vi "Get Test Limits File Path.vi"(6 "Lookup Table File Name":string="TestLimitsLookup.csv", 8 "error in (no error)":errorcluster, 9 "Filename Search Parameters":string, 10 "HW Version":dbl, 11 "Test Limits Directory":path) -> (0 "error out":errorcluster, 3 "Test Limits File Path":path)   [LabVIEW 2025, in "Test Limits.lvlib"]
uses:
  Test Limits.lvlib
  <vilib>/Utility/error.llb/Error Cluster From Error Code.vi
  <vilib>/ErrorRing/Error Ring.xnode
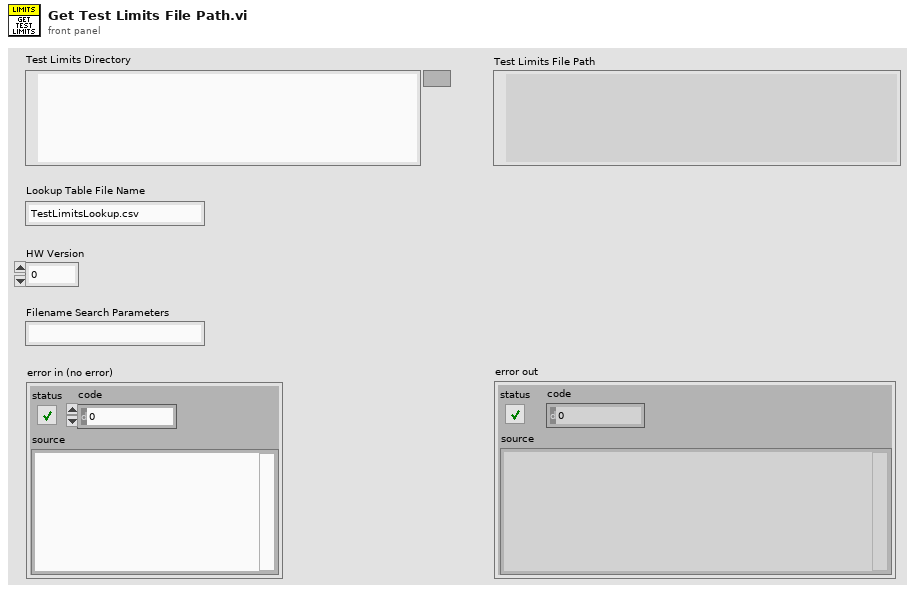
[diagram p1: front panel]
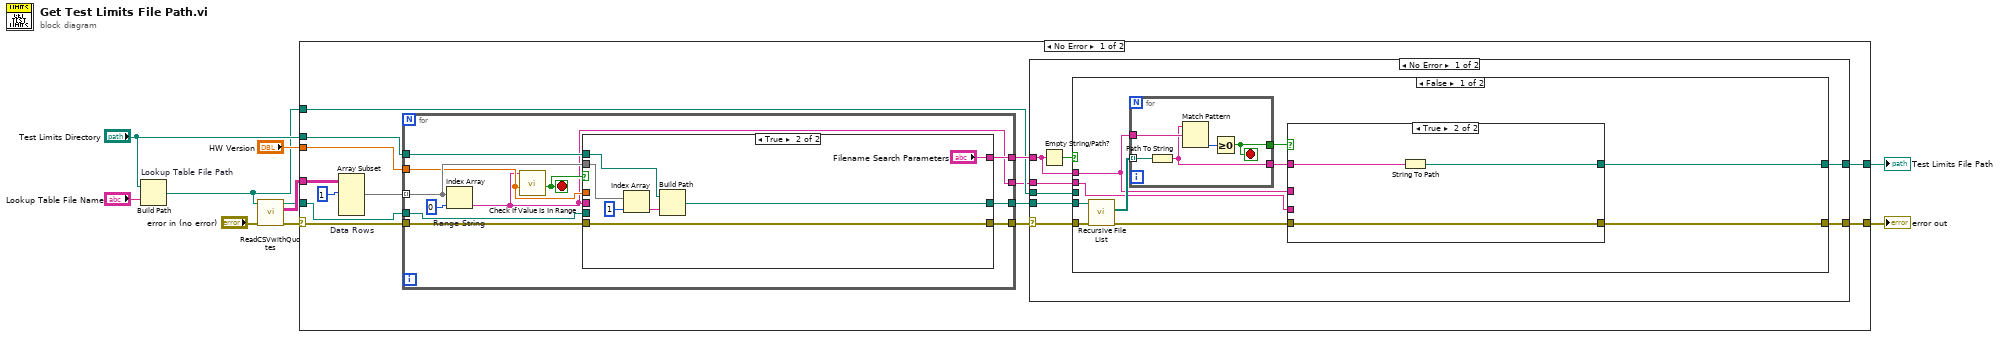
[diagram p0: block diagram]
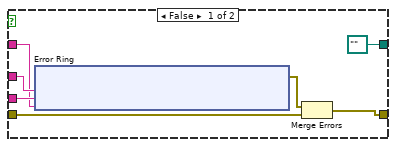
[diagram p2: hidden frame]
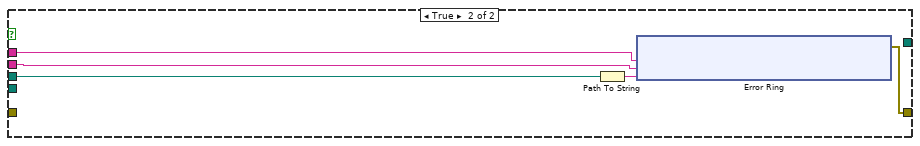
[diagram p3: hidden frame]
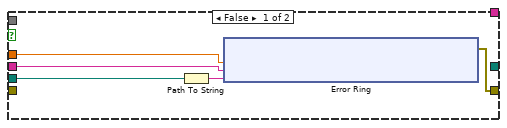
[diagram p5: hidden frame]
diagram:
  n1 = Build Path "Lookup Table File Path"(base path="Test Limits Directory", name or relative path="Lookup Table File Name") -> (appended path=w1:path)
  n2 = call "ReadCSVwithQuotes.vi"("error in (no error)"="error in (no error)", "File Path"=w1) -> ("error out"=w8:errorcluster, "Array"=w6:string[][], "File Path out"=w2:path)  [unwired: 7 in]
  n3 = case shown="No Error" w8 {
    selector: w8 -> [w22 w114]
    tunnel: [w17 w114] -> w7
    tunnel: w6 -> [w19 _]
    tunnel: "HW Version" -> [w21 _]
    tunnel: "Test Limits Directory" -> [w20 _]
    tunnel: [w15 _] -> w3
    tunnel: w2 -> [w14 _]
    tunnel: w1 -> [w12 _]
    frame No Error {
      n4 = Array Subset "Data Rows"(array=w19, index (row)=1 ("index")) -> (w23:string[][])  [unwired: 3 in]
      n5 = for {
        tunnel: w23 -> [w89] mode=indexing
        tunnel: w22 -> [w86]
        tunnel: [w85] -> w13
        tunnel: w21 -> [w83]
        tunnel: w20 -> [w90]
        tunnel: [w88] -> w18
        tunnel: [w87] -> w16
        tunnel: w14 -> [w84]
        tunnel: [w82] -> w11
        stop <- w91 stop-if-true
        n6 = Index Array "Range String"(array=w89, index=0) -> (element=w82:string)
        n7 = call "Check If Value Is In Range.vi"("Value"=w83, "Range String"=w82) -> ("In Range?"=w91:bool)  [unwired: 7 in, 2 out]
        n8 = case shown="True" w91 {
          tunnel: w90 -> [_ w113]
          tunnel: w89 -> [_ w109]
          tunnel: [_ w110] -> w88
          tunnel: [_ "Filename Search Parameters"] -> w87
          tunnel: w86 -> [_ w108]
          tunnel: [w93 w108] -> w85
          tunnel: w84 -> [w96 _]
          tunnel: w83 -> [w95 _]
          tunnel: w82 -> [w94 _]
          frame False {
            n9 = Path To String(path=w96) -> (string=w97:string)
            n10 = xnode "Error Ring"("parameter 0"=w95, "parameter 1"=w94, "parameter 2"=w97) -> ("error out"=w93:errorcluster)
          }
          frame True {
            n11 = Index Array(array=w109, index=1) -> (element=w111:string)
            n12 = Build Path(base path=w113, name or relative path=w111) -> (appended path=w110:path)
          }
        }
      }
      n13 = case shown="No Error" w13 {
        selector: w13 -> [w27 w81]
        tunnel: w18 -> [w31 _]
        tunnel: [w30 w81] -> w17
        tunnel: w16 -> [w29 _]
        tunnel: [w28 _] -> w15
        tunnel: w12 -> [w26 _]
        tunnel: w11 -> [w25 _]
        frame No Error {
          n14 = Empty String/Path?(string/path=w29) -> (empty?=w32:bool)
          n15 = case shown="False" w32 {
            tunnel: w31 -> [w42 _]
            tunnel: w27 -> [w41 _]
            tunnel: [w35 w68] -> w30
            tunnel: w29 -> [w34 w67]
            tunnel: [w38 _] -> w28
            tunnel: w26 -> [_ w70]
            tunnel: w25 -> [w33 w69]
            frame False {
              n16 = call <vilib>:"Recursive File List.vi"("error in (no error)"=w41, "Folder Path"=w42) -> ("error out"=w36:errorcluster, "All Files in Dir"=w40:path[])  [unwired: 5 in, 3 out]
              n17 = for {
                tunnel: w40 -> [w65] mode=indexing
                tunnel: w34 -> [w64]
                tunnel: [w63] -> w39
                tunnel: [w62] -> w37
                stop <- w62 stop-if-true
                n18 = Path To String(path=w65) -> (string=w63:string)
                n19 = Match Pattern(string=w63, regular expression=w64) -> (offset past match=w66:i32)  [unwired: 1 in, 3 out]
                n20 = Greater Or Equal To 0?(x=w66) -> (x >= 0?=w62:bool)
              }
              n21 = case shown="True" w37 {
                tunnel: w39 -> [w43 w61]
                tunnel: [path "" w60] -> w38
                tunnel: w36 -> [w47 w59]
                tunnel: [w46 w59] -> w35
                tunnel: w34 -> [w45 _]
                tunnel: w33 -> [w44 _]
                frame False {
                  n22 = xnode "Error Ring"("parameter 0"=w45, "parameter 1"=w44, "parameter 2"=w43) -> ("error out"=w48:errorcluster)
                  n23 = Merge Errors(w48, w47) -> (w46:errorcluster)
                }
                frame True {
                  n24 = String To Path(string=w61) -> (path=w60:path)
                }
              }
            }
            frame True {
              n25 = Path To String(path=w70) -> (string=w71:string)
              n26 = xnode "Error Ring"("parameter 0"=w67, "parameter 1"=w69, "parameter 2"=w71) -> ("error out"=w68:errorcluster)
            }
          }
        }
        frame Error {
        }
      }
    }
    frame Error {
    }
  }
  "error out" <- w7
  "Test Limits File Path" <- w3
